vi "Automated_measure.vi"(0 "VISA resource name":refnum<visa-resource-name>, 4 "file path (dialog if empty)":path, 5 "Samples per position":i32, 7 "error in":errorcluster, 9 "Baud rate (115200)":u32=115200 min=38400 max=500000 step=1, 11 "Import":path, 12 "Cal Param":sgl[](array[numeric]), 13 "Initial Tare":sgl[](array[numeric])) -> (1 "Measure":T1, 3 "Motor Ready":bool, 8 "VISA resource name out":refnum<visa-resource-name>, 10 "Communication OK":bool, 14 "Monitor":T2, 15 "error out":errorcluster)   [LabVIEW 2018]
uses:
  <vilib>/Utility/file.llb/Read Delimited Spreadsheet (DBL).vi
  Progress.vi
  <vilib>/Utility/file.llb/Write Delimited Spreadsheet (DBL).vi
panel:
  out "element":dbl
  out "Progress":u8(slide) scale=0.0..100.0
  # "%"
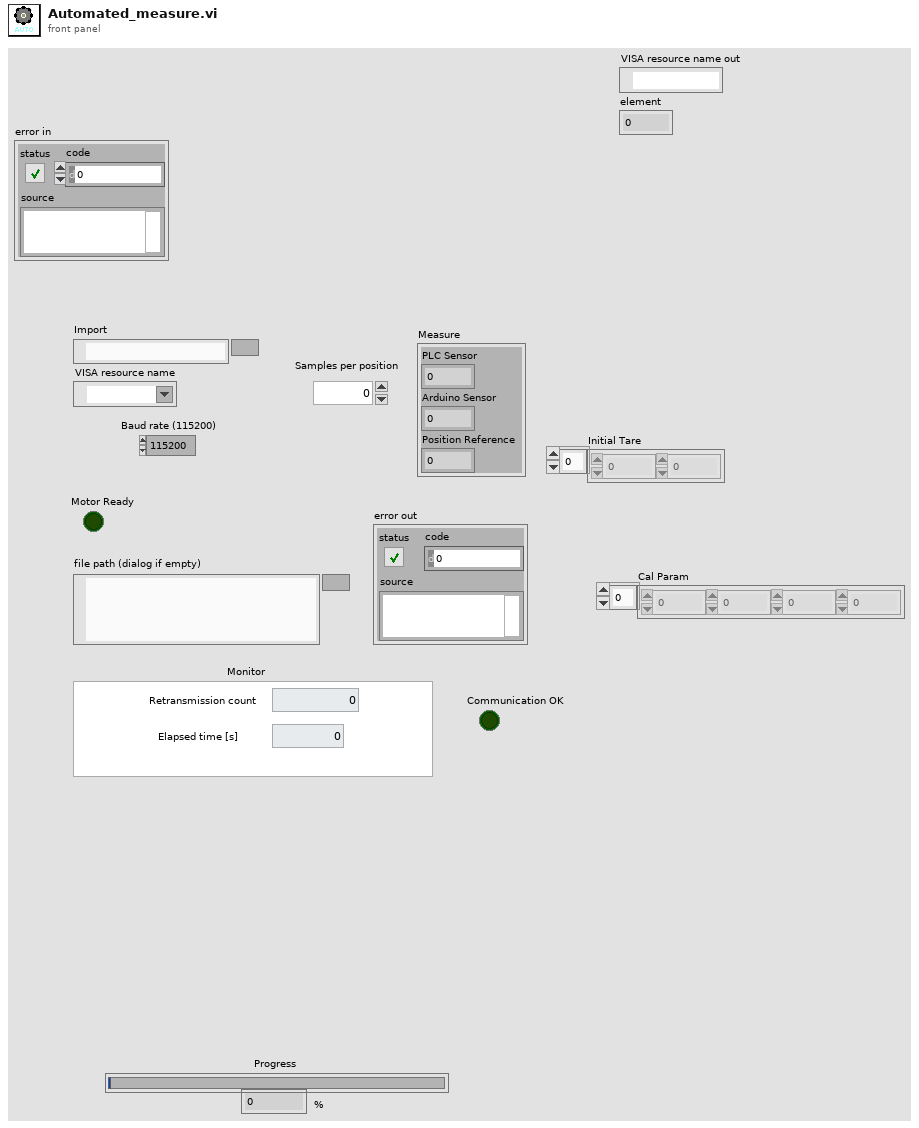
[diagram p1: front panel]
types:
  T1 = cluster{"PLC Sensor":dbl, "Arduino Sensor":dbl, "Position Reference":dbl}
  T2 = cluster{"Elapsed time [s]":dbl, "Retransmission count":dbl}
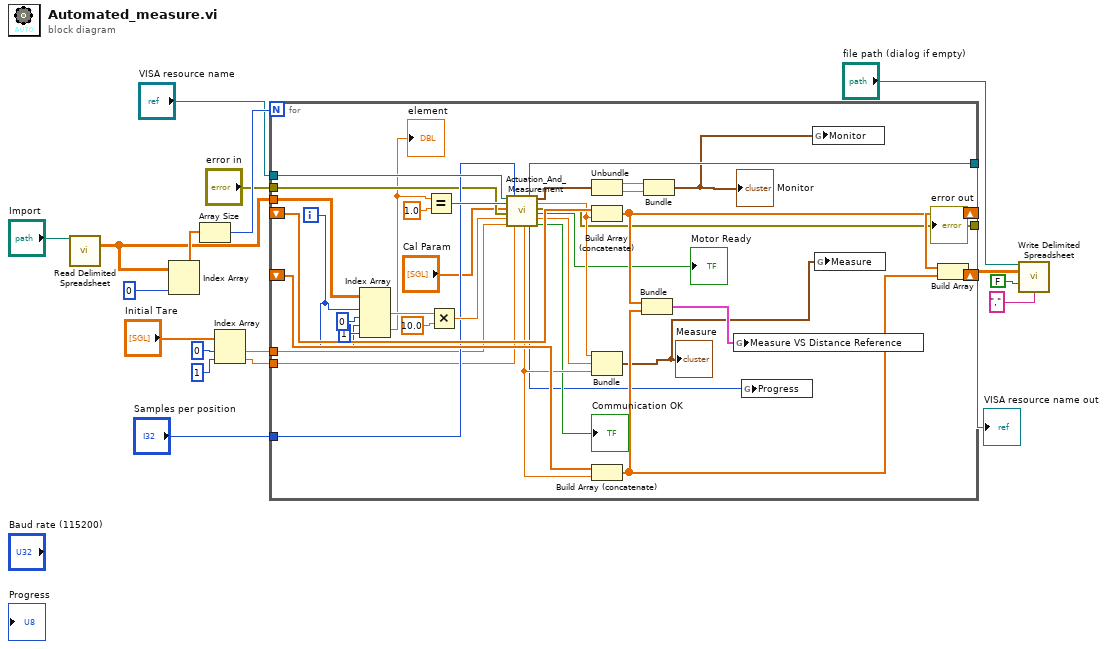
[diagram p0: block diagram]
diagram:
  n1 = call-poly <vilib>:"Read Delimited Spreadsheet.vi"("file path (dialog if empty)"="Import") -> ("all rows"=w1:dbl[][])  [unwired: 9 in, 5 out]
  n2 = Index Array(array=w1, index (col)=0 ("disabled index (col)")) -> (element=w19:dbl[])  [unwired: 1 in]
  n3 = Array Size(array=w19) -> (size(s)=w14:i32)
  n4 = Index Array(array="Initial Tare", index #1=0 ("index"), index #2=1 ("index")) -> (element #1=w6:sgl, element #2=w5:sgl)
  n5 = for {
    N: w14 -> [_]
    shift-right: [w53] -> w17
    shift-left: _ -> [w55]
    shift-right: [w52] -> w16
    shift-left: _ -> [w54]
    tunnel: [w40] -> w15
    tunnel: "VISA resource name" -> [w39]
    tunnel: w1 -> [w38]
    tunnel: "Samples per position" -> [w34]
    tunnel: "error in" -> [w33]
    tunnel: w6 -> [w31]
    tunnel: w5 -> [w30]
    tunnel: [w29] -> w2
    i -> [w25]
    n6 = Index Array(array=w38, index (row) #1=w25, index (col) #1=0 ("disabled index (col)"), index (row) #2=w25, index (col) #2=1 ("index (col)")) -> (element #1=w37:dbl, element #2=w26:dbl)
    "element" <- w26
    n7 = Equal?(x=w26, y=1.0) -> (x = y?=w47:bool)
    n8 = Multiply(x=w37, y=10.0) -> (x*y=w49:dbl)
    n9 = call "Actuation_And_Measurement.vi"("VISA resource name"=w39, "Direction"=w47, "Cal Param"="Cal Param", "error in (no error)"=w33, "Motor relative position"=w49, "Zero Offset"=w31, "Samples per position"=w34, "Fullscale"=w30) -> ("Position Reference"=w46:dbl, "VISA resource name out"=w29:refnum<visa-resource-name>, "Progress"=w28:u8, "Monitor"=w43:T2, "PLC Sensor"=w44:dbl, "error out"=w40:errorcluster, "Motor Ready"=→"Motor Ready":bool, "Arduino Sensor"=w45:dbl, "Communication\nAcknowledged"=→"Communication OK":bool)  [unwired: 2 in, 1 out]
    n10 = Unbundle(w43) -> ("Elapsed time [s]"=w42:dbl, "Retransmission count"=w41:dbl)
    n11 = Build Array (concatenate)(w55, w44) -> (w53:dbl[])
    n12 = Bundle("PLC Sensor"=w44, "Arduino Sensor"=w45, "Position Reference"=w46) -> (w22:T1)  [unwired: 1 in]
    "Measure" <- w22
    n13 = Build Array (concatenate)(w54, w46) -> (w52:dbl[])
    n14 = Bundle(w53, w52) -> (w24:cluster{dbl[], dbl[]})  [unwired: 1 in]
    n15 = Bundle("Elapsed time [s]"=w42, "Retransmission count"=w41) -> (w23:T2)  [unwired: 1 in]
    "Monitor" <- w23
    n16 = global write "Progress.vi" "Measure VS Distance Reference"(w24) -> ()
    n17 = global write "Progress.vi" "Progress"(w28) -> ()
    n18 = global write "Progress.vi" "Monitor"(w23) -> ()
    n19 = global write "Progress.vi" "Measure"(w22) -> ()
  }
  "error out" <- w15
  "VISA resource name out" <- w2
  n20 = Build Array(w17, w16) -> (w18:dbl[][])
  n21 = call-poly <vilib>:"Write Delimited Spreadsheet.vi"("file path (dialog if empty)"="file path (dialog if empty)", "2D data"=w18, "append to file? (new file:F)"=FALSE, "delimiter (\\t)"="," ("delimiter (\\t)")) -> ()  [unwired: 10 in, 2 out]
